vi "setLinear.vi"(5 "toFlash":bool, 6 "Error":bool, 7 "VISA resource name":refnum<visa-resource-name>="ASRL13::INSTR") -> (2 "Error":bool, 3 "dup VISA resource name":refnum<visa-resource-name>="ASRL13::INSTR")   [LabVIEW 2018]
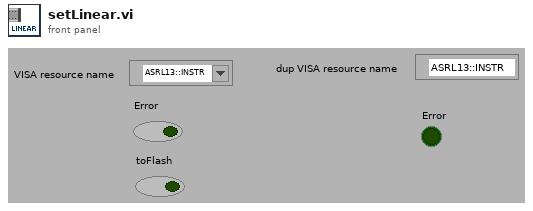
[diagram p1: front panel]
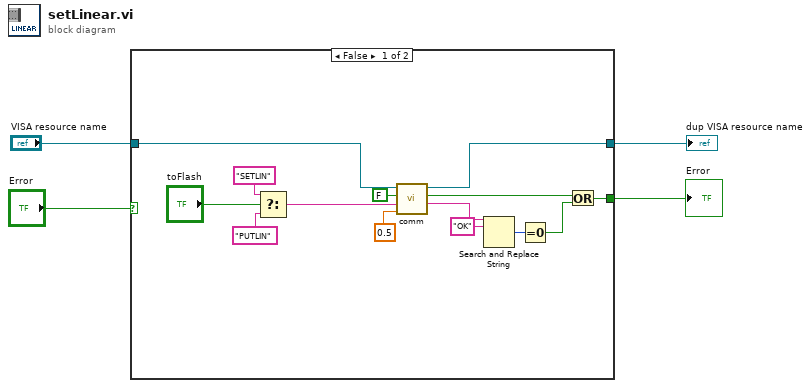
[diagram p0: block diagram]
diagram:
  n1 = case shown="False" "Error" {
    selector: "Error" -> [_ w20]
    tunnel: "VISA resource name" -> [w18 w19]
    tunnel: [w11 w20] -> w3
    tunnel: [w17 w19] -> w2
    frame False {
      n2 = Select(t="SETLIN" ("Substring"), s="toFlash", f="PUTLIN" ("Substring")) -> (s? t:f=w5:string)
      n3 = call "comm.vi"("Timeout (s)"=0.5, "Command"=w5, "Error"=FALSE, "VISA resource name"=w18) -> ("Response"=w14:string, "Error"=w10:bool, "dup VISA resource name"=w17:refnum<visa-resource-name>)  [unwired: 2 in, 1 out]
      n4 = Search and Replace String(input string=w14, search string="OK") -> (number of replacements=w12:i32)  [unwired: 6 in, 3 out]
      n5 = Equal To 0?(x=w12) -> (x = 0?=w9:bool)
      n6 = Or(x=w10, y=w9) -> (x .or. y?=w11:bool)
    }
    frame True {
    }
  }
  "Error" <- w3
  "dup VISA resource name" <- w2
